vi "StartUp Sequence Open Loop Rev 1.4.vi"() -> ()   [LabVIEW 2017]
panel:
  out "Waveform Chart":cluster{i32, i32}(graph)
  in  "Set Pump Value 1":string
  out "Pump Value 2":string
  in  "Soft Shut Off":bool
  out "Pump Value 1":string
  in  "Send Pump":bool
  in  "Send Command":bool
  in  "Custom Command":string
  out "Startup Success":bool
  in  "Output File":path
  in  "Shut Off":bool
  out "ECU COM Port Out":refnum<visa-resource-name>
  out "Throttle Position":string
  out "Turbine RPM":string
  out "Turbine Temp":string
  out "Error Out":errorcluster
  in  "Error In":errorcluster
  in  "ECU COM Port":refnum<visa-resource-name>
  out "Turbine State":string
  in  "Strt Sqnc":bool
  # "Note: save to a .csv file"
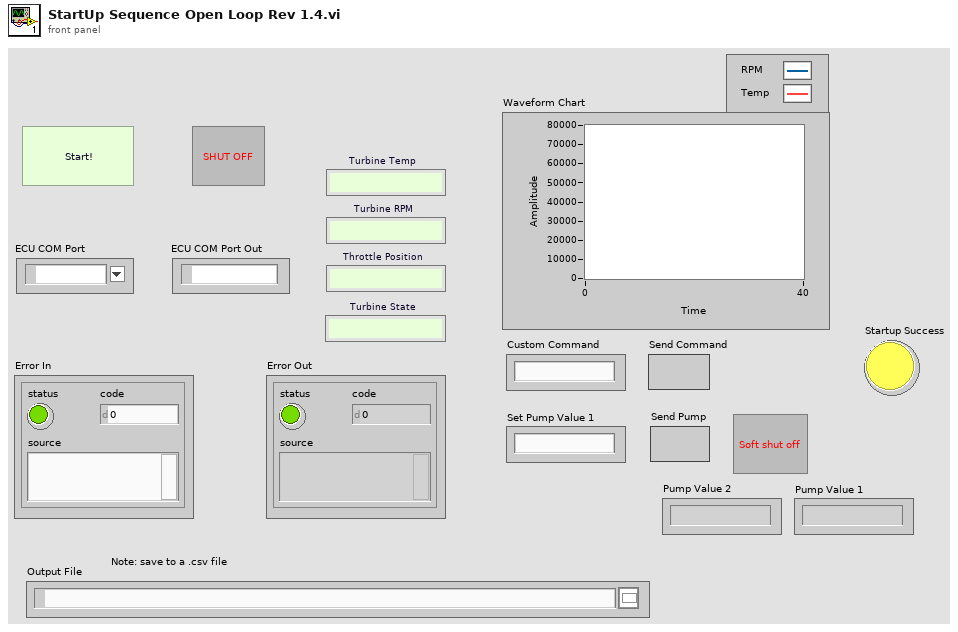
[diagram p1: front panel]
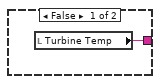
[diagram p4: hidden frame]
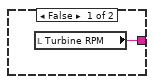
[diagram p5: hidden frame]
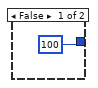
[diagram p7: hidden frame]
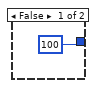
[diagram p8: hidden frame]
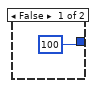
[diagram p9: hidden frame]
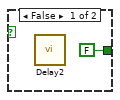
[diagram p11: hidden frame]
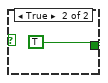
[diagram p12: hidden frame]
diagram:
  w7 = 21 ("Pulse Width")
  w8 = 160 ("Voltage")
  w13 = 16 ("Pulse Width")
  w14 = 160 ("Voltage")
  w4 = 255 ("y")
  w5 = 80 ("y")
  # "Disengage Starter Motor"
  # "Starter Motor 55%"
  # "Start button is inside a while loop that doesn't progess until True"
  # "Fuel Pump Mode 2"
  # "GlowPlugOff"
  # "Start Up\nFuelPumpMode 1"
  # "BurnerValveIgnitionPercent"
  # "If False, each Case structure is set\nto an arbitrary Delay time of 0.2 s"
  # "Each Stage is inside a while loop so that \nthe sequence doesn't progress until True"
  n1 = call "Initialize Com Port.vi"("Error In"="Error In", "ECU COM Port"="ECU COM Port") -> ("Error Out"=w28:errorcluster, "ECU COM Port Out"=w27:refnum<visa-resource-name>)  [unwired: 8 in]
  n2 = while {
    tunnel: w28 -> [w125]
    tunnel: [w125] -> w26
    stop <- "Strt Sqnc" stop-if-true
  }
  n3 = call "Initialize Output File.vi"("error in (no error)"=w26, "File Path Control"="Output File") -> ("error out"=w3:errorcluster)  [unwired: 9 in]
  n4 = flat-sequence {
    tunnel: w3 -> [w127]
    tunnel: [w127] -> w18
    frame #0 {
      n5 = local write "Strt Sqnc"(FALSE ("Strt Sqnc")) -> ()
    }
  }
  n6 = flat-sequence {
    tunnel: [w130] -> w2
    tunnel: w3 -> [w130]
    frame #0 {
      w129 = "0" ("Pump Value 1")
      n7 = local write "Pump Value 2"(w129) -> ()
      n8 = local write "Pump Value 1"(w129) -> ()
    }
  }
  n9 = while {
    tunnel: w2 -> [w151]
    tunnel: w27 -> [w150]
    tunnel: "Output File" -> [w147]
    stop <- w146 continue-if-true
    n10 = call "Get Engine Update.vi"("Error In"=w151, "ECU COM Port"=w150) -> ("Error Out"=w148:errorcluster, "Temperature"=w139:string, "RPMs"=w143:string, "ECU COM Port Out"=w145:refnum<visa-resource-name>)  [unwired: 6 in]
    n11 = call "Time Delay4"() -> ()  [unwired: 11 in, 1 out]
    n12 = call "Safety Check.vi"("Temperature"=w139, "RPMs"=w143) -> ("Safe?"=w146:bool)  [unwired: 9 in]
    n13 = Not Equal?(x=w143, y="") -> (x != y?=w141:bool)
    n14 = Not Equal?(x=w139, y="") -> (x != y?=w138:bool)
    n15 = case shown="False" w146 {
      selector: w146 -> [w156 w158]
      tunnel: w145 -> [w157 _]
      tunnel: [w156 w158] -> w144
      frame False {
        n16 = call "Emergency Shutoff.vi"("ECU COM Port"=w157) -> ()  [unwired: 9 in, 2 out]
      }
      frame True {
      }
    }
    n17 = case shown="True" w141 {
      tunnel: w143 -> [_ w155]
      tunnel: [w154 w155] -> w134
      frame False {
        n18 = local read "Turbine RPM"() -> (w154:string)
      }
      frame True {
        "Turbine RPM" <- w155
      }
    }
    n19 = case shown="True" w138 {
      tunnel: w139 -> [_ w153]
      tunnel: [w152 w153] -> w133
      frame False {
        n20 = local read "Turbine Temp"() -> (w152:string)
      }
      frame True {
        "Turbine Temp" <- w153
      }
    }
    n21 = Not(x=w144) -> (.not. x?=w149:bool)
    n22 = Stop(stop? (T)=w149) -> ()
    n23 = local read "Pump Value 2"() -> (w136:string)
    n24 = local read "Pump Value 1"() -> (w137:string)
    n25 = Decimal String To Number(string=w134) -> (number=w131:i32)  [unwired: 2 in, 1 out]
    n26 = Decimal String To Number(string=w133) -> (number=w132:i32)  [unwired: 2 in, 1 out]
    n27 = Bundle(w131, w132) -> (→"Waveform Chart":cluster{i32, i32})  [unwired: 1 in]
    n28 = call "Write Data to Output File.vi"("Pump Value 2"=w136, "Pump Value 1"=w137, "Error In"=w148, "Temperature"=w133, "RPM"=w134, "File Path Control"=w147) -> ()  [unwired: 5 in, 1 out]
  }
  n29 = while {
    tunnel: w27 -> [w160]
    tunnel: w28 -> [_]
    stop <- FALSE stop-if-true
    n30 = case shown="True" "Send Command" {
      tunnel: "Custom Command" -> [_ w164]
      tunnel: w160 -> [_ w163]
      frame False {
      }
      frame True {
        n31 = call "Time Delay3"() -> ()  [unwired: 11 in, 1 out]
        n32 = VISA Write(VISA resource name=w163, write buffer=w164) -> ()  [unwired: 1 in, 3 out]
      }
    }
  }
  n33 = flat-sequence {
    tunnel: w18 -> [_]
    frame #0 {
      n34 = local write "Turbine State"("Initializing Motor") -> ()
    }
  }
  n35 = while {
    tunnel: ["Shut Off"] -> w122
    tunnel: "ECU COM Port" -> [w166]
    stop <- "Shut Off" stop-if-true
    # "Turns off each individual component"
    n36 = case shown="True" "Shut Off" {
      tunnel: w166 -> [_ w170]
      frame False {
      }
      frame True {
        n37 = call "Emergency Shutoff.vi"("ECU COM Port"=w170) -> ("Error Out"=w169:errorcluster)  [unwired: 9 in, 1 out]
        n38 = local write "Output File"(path "" ("Output File")) -> ()
        n39 = flat-sequence {
          tunnel: w169 -> [w171]
          tunnel: [w171] -> _
          frame #0 {
            n40 = local write "Strt Sqnc"(FALSE ("Strt Sqnc")) -> ()
          }
        }
      }
    }
  }
  n41 = call "Set Glow Plug Duty Cycle.vi"("Error In"=w18, "Duty Cycle"=6, "ECU COM Port"=w27) -> ("Error Out"=w113:errorcluster, "ECU COM Port Out"=w110:refnum<visa-resource-name>)  [unwired: 7 in]
  n42 = call "Delay"("error in (no error)"=w113) -> ("error out"=w112:errorcluster)  [unwired: 10 in]
  n43 = call "Set Glow Plug Duty Cycle.vi"("Error In"=w112, "Duty Cycle"=19, "ECU COM Port"=w110) -> ("Error Out"=w111:errorcluster, "ECU COM Port Out"=w106:refnum<visa-resource-name>)  [unwired: 7 in]
  n44 = call "Delay"("error in (no error)"=w111) -> ("error out"=w107:errorcluster)  [unwired: 10 in]
  n45 = call "Set Starter Motor Duty Cycle.vi"("Error In"=w107, "Duty Cycle"=6, "ECU COM Port"=w106) -> ("Error Out"=w105:errorcluster, "ECU COM Port Out"=w103:refnum<visa-resource-name>)  [unwired: 7 in]
  n46 = call "Set Glow Plug Duty Cycle.vi"("Error In"=w105, "Duty Cycle"=15, "ECU COM Port"=w103) -> ("Error Out"=w104:errorcluster, "ECU COM Port Out"=w99:refnum<visa-resource-name>)  [unwired: 7 in]
  n47 = call "Delay"("error in (no error)"=w104) -> ("error out"=w101:errorcluster)  [unwired: 10 in]
  n48 = call "Set Starter Motor Duty Cycle.vi"("Error In"=w101, "Duty Cycle"=4, "ECU COM Port"=w99) -> ("Error Out"=w100:errorcluster, "ECU COM Port Out"=w98:refnum<visa-resource-name>)  [unwired: 7 in]
  n49 = call "Delay"("error in (no error)"=w100) -> ("error out"=w123:errorcluster)  [unwired: 10 in]
  n50 = Stop(stop? (T)=w122) -> ()
  n51 = while {
    tunnel: w123 -> [w175]
    tunnel: w98 -> [w174]
    tunnel: [w174] -> w16
    tunnel: [w175] -> w124
    stop <- w178 stop-if-true
    n52 = local read "Turbine RPM"() -> (w173:string)
    n53 = Decimal String To Number(string=w173) -> (number=w177:i32)  [unwired: 2 in, 1 out]
    n54 = Greater Or Equal?(x=w177, y=3300) -> (x >= y?=w179:bool)
    n55 = case shown="True" w179 {
      tunnel: [FALSE TRUE] -> w178
      frame False {
        n56 = call "Delay2"() -> ()  [unwired: 11 in, 1 out]
      }
      frame True {
      }
    }
  }
  n57 = flat-sequence {
    tunnel: w123 -> [_]
    frame #0 {
      n58 = local write "Turbine State"("Stage1 Check RPM") -> ()
    }
  }
  n59 = call "CmdSeparator7"("error in (no error)"=w124) -> ("error out"=w12:errorcluster)  [unwired: 10 in]
  n60 = call "Set Pump Fow Rate.vi"("Error In"=w12, "Pulse Width"=w13, "Voltage"=w14, "ECU COM Port"=w16) -> ("Error Out"=w17:errorcluster, "ECU COM Port Out"=w15:refnum<visa-resource-name>)  [unwired: 6 in]
  n61 = flat-sequence {
    tunnel: w14 -> [w184]
    tunnel: w13 -> [w183]
    tunnel: w12 -> [_]
    frame #0 {
      n62 = Number To Decimal String(number=w183) -> (decimal integer string=w185:string)  [unwired: 1 in]
      n63 = Number To Decimal String(number=w184) -> (decimal integer string=w186:string)  [unwired: 1 in]
      n64 = local write "Pump Value 2"(w185) -> ()
      n65 = local write "Pump Value 1"(w186) -> ()
    }
  }
  n66 = call "CmdSeparator2"("error in (no error)"=w17) -> ("error out"=w97:errorcluster)  [unwired: 10 in]
  n67 = call "Set Burner Valve Percent.vi"("Error In"=w97, "Percent"=10, "ECU COM Port"=w15) -> ("Error Out"=w96:errorcluster, "ECU COM Port Out"=w86:refnum<visa-resource-name>)  [unwired: 7 in]
  n68 = call "CmdSeparator"("error in (no error)"=w96) -> ("error out"=w95:errorcluster)  [unwired: 10 in]
  n69 = call "Set Burner Valve Percent.vi"("Error In"=w95, "Percent"=31, "ECU COM Port"=w86) -> ("Error Out"=w94:errorcluster, "ECU COM Port Out"=w85:refnum<visa-resource-name>)  [unwired: 7 in]
  n70 = call "CmdSeparator10"("error in (no error)"=w94) -> ("error out"=w93:errorcluster)  [unwired: 10 in]
  n71 = call "Set Burner Valve Percent.vi"("Error In"=w93, "Percent"=35, "ECU COM Port"=w85) -> ("Error Out"=w92:errorcluster, "ECU COM Port Out"=w84:refnum<visa-resource-name>)  [unwired: 7 in]
  n72 = call "CmdSeparator11"("error in (no error)"=w92) -> ("error out"=w91:errorcluster)  [unwired: 10 in]
  n73 = call "Set Burner Valve Percent.vi"("Error In"=w91, "Percent"=39, "ECU COM Port"=w84) -> ("Error Out"=w90:errorcluster, "ECU COM Port Out"=w83:refnum<visa-resource-name>)  [unwired: 7 in]
  n74 = call "CmdSeparator12"("error in (no error)"=w90) -> ("error out"=w89:errorcluster)  [unwired: 10 in]
  n75 = call "Set Burner Valve Percent.vi"("Error In"=w89, "Percent"=43, "ECU COM Port"=w83) -> ("Error Out"=w88:errorcluster, "ECU COM Port Out"=w82:refnum<visa-resource-name>)  [unwired: 7 in]
  n76 = call "CmdSeparator13"("error in (no error)"=w88) -> ("error out"=w87:errorcluster)  [unwired: 10 in]
  n77 = call "Set Burner Valve Percent.vi"("Error In"=w87, "Percent"=47, "ECU COM Port"=w82) -> ("Error Out"=w65:errorcluster, "ECU COM Port Out"=w64:refnum<visa-resource-name>)  [unwired: 7 in]
  n78 = call "CmdSeparator6"("error in (no error)"=w65) -> ("error out"=w67:errorcluster)  [unwired: 10 in]
  n79 = call "Set Burner Valve Percent.vi"("Error In"=w67, "Percent"=51, "ECU COM Port"=w64) -> ("Error Out"=w60:errorcluster, "ECU COM Port Out"=w61:refnum<visa-resource-name>)  [unwired: 7 in]
  n80 = call "CmdSeparator8"("error in (no error)"=w60) -> ("error out"=w63:errorcluster)  [unwired: 10 in]
  n81 = call "Set Burner Valve Percent.vi"("Error In"=w63, "Percent"=55, "ECU COM Port"=w61) -> ("Error Out"=w56:errorcluster, "ECU COM Port Out"=w57:refnum<visa-resource-name>)  [unwired: 7 in]
  n82 = call "CmdSeparator14"("error in (no error)"=w56) -> ("error out"=w59:errorcluster)  [unwired: 10 in]
  n83 = call "Set Burner Valve Percent.vi"("Error In"=w59, "Percent"=59, "ECU COM Port"=w57) -> ("Error Out"=w55:errorcluster, "ECU COM Port Out"=w54:refnum<visa-resource-name>)  [unwired: 7 in]
  n84 = call "CmdSeparator9"("error in (no error)"=w55) -> ("error out"=w121:errorcluster)  [unwired: 10 in]
  n85 = flat-sequence {
    tunnel: w121 -> [_]
    frame #0 {
      n86 = local write "Turbine State"("Stage2 Check Temp.") -> ()
    }
  }
  n87 = while {
    tunnel: w54 -> [w189]
    tunnel: w121 -> [w190]
    tunnel: [w189] -> w71
    tunnel: [w190] -> w72
    stop <- w193 stop-if-true
    # "Stage2Temp(C)"
    n88 = local read "Turbine Temp"() -> (w188:string)
    n89 = Decimal String To Number(string=w188) -> (number=w191:i32)  [unwired: 2 in, 1 out]
    n90 = Greater Or Equal?(x=w191, y=90) -> (x >= y?=w194:bool)
    n91 = case shown="False" w194 {
      tunnel: [FALSE TRUE] -> w193
      frame False {
        n92 = call "Delay3"() -> ()  [unwired: 11 in, 1 out]
      }
      frame True {
      }
    }
  }
  n93 = call "Set Glow Plug Duty Cycle.vi"("Error In"=w72, "Duty Cycle"=0, "ECU COM Port"=w71) -> ("Error Out"=w70:errorcluster, "ECU COM Port Out"=w9:refnum<visa-resource-name>)  [unwired: 7 in]
  n94 = call "CmdSeparator3"("error in (no error)"=w70) -> ("error out"=w6:errorcluster)  [unwired: 10 in]
  n95 = call "Set Pump Fow Rate.vi"("Error In"=w6, "Pulse Width"=w7, "Voltage"=w8, "ECU COM Port"=w9) -> ("Error Out"=w11:errorcluster, "ECU COM Port Out"=w10:refnum<visa-resource-name>)  [unwired: 6 in]
  n96 = call "Set Burner Valve Percent.vi"("Error In"=w11, "Percent"=80, "ECU COM Port"=w10) -> ("Error Out"=w53:errorcluster, "ECU COM Port Out"=w68:refnum<visa-resource-name>)  [unwired: 7 in]
  n97 = flat-sequence {
    tunnel: w8 -> [w198]
    tunnel: w7 -> [w197]
    tunnel: w6 -> [_]
    frame #0 {
      n98 = Number To Decimal String(number=w197) -> (decimal integer string=w199:string)  [unwired: 1 in]
      n99 = Number To Decimal String(number=w198) -> (decimal integer string=w200:string)  [unwired: 1 in]
      n100 = local write "Pump Value 2"(w199) -> ()
      n101 = local write "Pump Value 1"(w200) -> ()
    }
  }
  n102 = call "CmdSeparator18"("error in (no error)"=w53) -> ("error out"=w52:errorcluster)  [unwired: 10 in]
  n103 = call "Set Fuel Valve Percent.vi"("Error In"=w52, "Percent"=12, "ECU COM Port"=w68) -> ("Error Out"=w51:errorcluster, "ECU COM Port Out"=w69:refnum<visa-resource-name>)  [unwired: 7 in]
  n104 = call "CmdSeparator16"("error in (no error)"=w51) -> ("error out"=w119:errorcluster)  [unwired: 10 in]
  n105 = for {
    N: 4 -> [_]
    tunnel: [w201] -> _
    tunnel: [w215] -> _
    tunnel: w69 -> [w207]
    tunnel: w119 -> [w208]
    shift-right: [w206] -> w47
    shift-left: 12 -> [w212]
    shift-right: [w203] -> _
    shift-left: 80 -> [w209]
    tunnel: [w215] -> w42 mode=indexing
    tunnel: [w201] -> w48 mode=indexing
    n106 = Less?(x=w212, y=100) -> (x < y?=w213:bool)
    n107 = Less?(x=w209, y=100) -> (x < y?=w210:bool)
    n108 = case shown="True" w210 {
      tunnel: w209 -> [_ w219]
      tunnel: [100 w217] -> w203
      frame False {
      }
      frame True {
        n109 = Add(x=w219, y=5) -> (x+y=w217:i32)
      }
    }
    n110 = case shown="True" w213 {
      tunnel: w212 -> [_ w223]
      tunnel: [100 w221] -> w206
      frame False {
      }
      frame True {
        n111 = Add(x=w223, y=6) -> (x+y=w221:i32)
      }
    }
    n112 = call "Set Fuel Valve Percent.vi"("Error In"=w208, "Percent"=w206, "ECU COM Port"=w207) -> ("Error Out"=w205:errorcluster, "ECU COM Port Out"=w202:refnum<visa-resource-name>)  [unwired: 7 in]
    n113 = call "Set Burner Valve Percent.vi"("Error In"=w205, "Percent"=w203, "ECU COM Port"=w202) -> ("Error Out"=w204:errorcluster, "ECU COM Port Out"=w201:refnum<visa-resource-name>)  [unwired: 7 in]
    n114 = call "CmdSeparator17"("error in (no error)"=w204) -> ("error out"=w215:errorcluster)  [unwired: 10 in]
  }
  n115 = flat-sequence {
    tunnel: w42 -> [_]
    frame #0 {
      n116 = local write "Turbine State"("Pump Ramp Up") -> ()
    }
  }
  n117 = for {
    N: 10 -> [_]
    tunnel: [w231] -> w30
    tunnel: [w242] -> w33
    shift-right: [w238] -> _
    shift-left: w47 -> [w239]
    tunnel: w42 -> [w235] mode=indexing
    tunnel: w48 -> [w234] mode=indexing
    shift-right: [w227] -> w44
    shift-left: 21 -> [w228]
    w226 = 160 ("y")
    n118 = Less?(x=w239, y=100) -> (x < y?=w240:bool)
    n119 = Add(x=w228, y=1) -> (x+y=w227:i32)
    n120 = case shown="True" w240 {
      tunnel: w239 -> [_ w250]
      tunnel: [100 w248] -> w238
      frame False {
      }
      frame True {
        n121 = Add(x=w250, y=5) -> (x+y=w248:i32)
      }
    }
    n122 = call "Set Fuel Valve Percent.vi"("Error In"=w235, "Percent"=w238, "ECU COM Port"=w234) -> ("Error Out"=w237:errorcluster, "ECU COM Port Out"=w236:refnum<visa-resource-name>)  [unwired: 7 in]
    n123 = call "Set Burner Valve Percent.vi"("Error In"=w237, "Percent"=100 ("y"), "ECU COM Port"=w236) -> ("Error Out"=w225:errorcluster, "ECU COM Port Out"=w232:refnum<visa-resource-name>)  [unwired: 7 in]
    n124 = call "Set Pump Fow Rate.vi"("Error In"=w225, "Pulse Width"=w227, "Voltage"=w226, "ECU COM Port"=w232) -> ("Error Out"=w230:errorcluster, "ECU COM Port Out"=w231:refnum<visa-resource-name>)  [unwired: 6 in]
    n125 = flat-sequence {
      tunnel: w226 -> [w244]
      tunnel: w227 -> [w243]
      tunnel: w225 -> [_]
      frame #0 {
        n126 = Number To Decimal String(number=w243) -> (decimal integer string=w245:string)  [unwired: 1 in]
        n127 = Number To Decimal String(number=w244) -> (decimal integer string=w246:string)  [unwired: 1 in]
        n128 = local write "Pump Value 2"(w245) -> ()
        n129 = local write "Pump Value 1"(w246) -> ()
      }
    }
    n130 = call "CmdSeparator20"("error in (no error)"=w230) -> ("error out"=w242:errorcluster)  [unwired: 10 in]
  }
  n131 = call "Set Starter Motor Duty Cycle.vi"("Error In"=w33, "Duty Cycle"=11, "ECU COM Port"=w30) -> ("Error Out"=w32:errorcluster, "ECU COM Port Out"=w31:refnum<visa-resource-name>)  [unwired: 7 in]
  n132 = flat-sequence {
    tunnel: w32 -> [_]
    frame #0 {
      n133 = local write "Turbine State"("Secondary Pump Ramp Up") -> ()
    }
  }
  n134 = for {
    N: 3 -> [_]
    tunnel: [w259] -> w43
    tunnel: [w266] -> w41
    tunnel: w32 -> [w263]
    tunnel: w31 -> [w262]
    shift-right: [w253] -> _
    shift-left: w44 -> [w256]
    w254 = 160 ("y")
    n135 = Add(x=w256, y=10) -> (x+y=w253:i32)
    n136 = call "Set Fuel Valve Percent.vi"("Error In"=w263, "Percent"=100 ("y"), "ECU COM Port"=w262) -> ("Error Out"=w265:errorcluster, "ECU COM Port Out"=w264:refnum<visa-resource-name>)  [unwired: 7 in]
    n137 = call "Set Burner Valve Percent.vi"("Error In"=w265, "Percent"=0 ("y"), "ECU COM Port"=w264) -> ("Error Out"=w252:errorcluster, "ECU COM Port Out"=w260:refnum<visa-resource-name>)  [unwired: 7 in]
    n138 = call "Set Pump Fow Rate.vi"("Error In"=w252, "Pulse Width"=w253, "Voltage"=w254, "ECU COM Port"=w260) -> ("Error Out"=w258:errorcluster, "ECU COM Port Out"=w259:refnum<visa-resource-name>)  [unwired: 6 in]
    n139 = flat-sequence {
      tunnel: w254 -> [w268]
      tunnel: w253 -> [w267]
      tunnel: w252 -> [_]
      frame #0 {
        n140 = Number To Decimal String(number=w267) -> (decimal integer string=w269:string)  [unwired: 1 in]
        n141 = Number To Decimal String(number=w268) -> (decimal integer string=w270:string)  [unwired: 1 in]
        n142 = local write "Pump Value 2"(w269) -> ()
        n143 = local write "Pump Value 1"(w270) -> ()
      }
    }
    n144 = call "CmdSeparator15"("error in (no error)"=w258) -> ("error out"=w266:errorcluster)  [unwired: 10 in]
  }
  n145 = flat-sequence {
    tunnel: w41 -> [_]
    frame #0 {
      n146 = local write "Turbine State"("Hold on to your butts!") -> ()
    }
  }
  n147 = while {
    tunnel: w41 -> [w273]
    tunnel: w43 -> [w272]
    tunnel: [w273] -> w1
    tunnel: [w272] -> w40
    stop <- w274 stop-if-true
    n148 = local read "Turbine RPM"() -> (w277:string)
    n149 = Decimal String To Number(string=w277) -> (number=w276:i32)  [unwired: 2 in, 1 out]
    n150 = Greater?(x=w276, y=30000) -> (0:w274:bool)
  }
  n151 = call "Set Pump Fow Rate.vi"("Error In"=w1, "Pulse Width"=w4, "Voltage"=w5, "ECU COM Port"=w40) -> ("Error Out"=w39:errorcluster, "ECU COM Port Out"=w38:refnum<visa-resource-name>)  [unwired: 6 in]
  n152 = flat-sequence {
    tunnel: w5 -> [w280]
    tunnel: w4 -> [w279]
    tunnel: [w278] -> _
    tunnel: w1 -> [w278]
    frame #0 {
      n153 = Number To Decimal String(number=w279) -> (decimal integer string=w281:string)  [unwired: 1 in]
      n154 = Number To Decimal String(number=w280) -> (decimal integer string=w282:string)  [unwired: 1 in]
      n155 = local write "Pump Value 2"(w281) -> ()
      n156 = local write "Pump Value 1"(w282) -> ()
    }
  }
  n157 = while {
    tunnel: w39 -> [w284]
    tunnel: w38 -> [w283]
    tunnel: [w284] -> w35
    tunnel: [w283] -> w37
    stop <- w285 stop-if-true
    n158 = local read "Turbine RPM"() -> (w288:string)
    n159 = Decimal String To Number(string=w288) -> (number=w287:i32)  [unwired: 2 in, 1 out]
    n160 = Greater?(x=w287, y=44000) -> (0:w285:bool)
  }
  n161 = flat-sequence {
    tunnel: w35 -> [_]
    frame #0 {
      n162 = local write "Turbine State"("Acheived Idle RPM!") -> ()
    }
  }
  n163 = call "Set Starter Motor Duty Cycle.vi"("Error In"=w35, "Duty Cycle"=0, "ECU COM Port"=w37) -> ("Error Out"=w24:errorcluster, "ECU COM Port Out"=w23:refnum<visa-resource-name>)  [unwired: 7 in]
  n164 = flat-sequence {
    tunnel: w24 -> [_]
    frame #0 {
      "Startup Success" <- TRUE
    }
  }
  n165 = while {
    tunnel: w23 -> [w303]
    tunnel: [w302] -> w21
    tunnel: [w301] -> w22
    tunnel: w24 -> [w299]
    stop <- "Soft Shut Off" stop-if-true
    n166 = Decimal String To Number(string="Set Pump Value 1") -> (number=w300:i32)  [unwired: 2 in, 1 out]
    n167 = Less?(x=w300, y=255) -> (x < y?=w295:bool)
    n168 = Greater Than 0?(x=w300) -> (x > 0?=w296:bool)
    n169 = And(x=w296, y=w295) -> (x .and. y?=w293:bool)
    n170 = call "Time Delay"() -> ()  [unwired: 11 in, 1 out]
    n171 = And(x=w293, y="Send Pump") -> (x .and. y?=w291:bool)
    n172 = case shown="True" w291 {
      tunnel: w303 -> [w304 w313]
      tunnel: w299 -> [w305 w312]
      tunnel: [w304 w311] -> w302
      tunnel: [w305 w310] -> w301
      tunnel: w300 -> [_ w307]
      frame False {
      }
      frame True {
        n173 = call "Set Pump Fow Rate.vi"("Error In"=w312, "Pulse Width"=255, "Voltage"=w307, "ECU COM Port"=w313) -> ("Error Out"=w310:errorcluster, "ECU COM Port Out"=w311:refnum<visa-resource-name>)  [unwired: 6 in]
        n174 = Number To Decimal String(number=w307) -> (decimal integer string=→"Pump Value 1":string)  [unwired: 1 in]
        n175 = local write "Pump Value 2"("255" ("Pump Value 2")) -> ()
      }
    }
  }
  n176 = call "Emergency Shutoff.vi"("Error In"=w22, "ECU COM Port"=w21) -> ("Error Out"=w20:errorcluster, "ECU COM Port Out"=→"ECU COM Port Out":refnum<visa-resource-name>)  [unwired: 8 in]
  n177 = flat-sequence {
    tunnel: w20 -> [w314]
    tunnel: [w314] -> w120
    frame #0 {
    }
  }
  "Error Out" <- w120
